vi "PMD Settings.vi"(0 "Visa In":refnum<visa-resource-name>, 1 "Zero?":refnum<vi>, 2 "PMD Settings In":T1 {"Averaging Rate" min=33 max=5000 step=1; "BWIn" items=["HIGH", "LOW"]; "Beam\nDiameter (mm)" min=1.0 max=9.0 step=0.5}, 3 "Error In":errorcluster, 4 "Range":i16 min=1 max=6 step=1) -> (5 "AUTO?":bool, 6 "Rng":string, 7 "Visa Out":refnum<visa-resource-name>, 8 "ZeroValue":dbl, 9 "PM Error log":string, 10 "error out":errorcluster)   [LabVIEW 2009]
panel:
  out "RANG_Val":dbl
  out "RANG_lbl":string
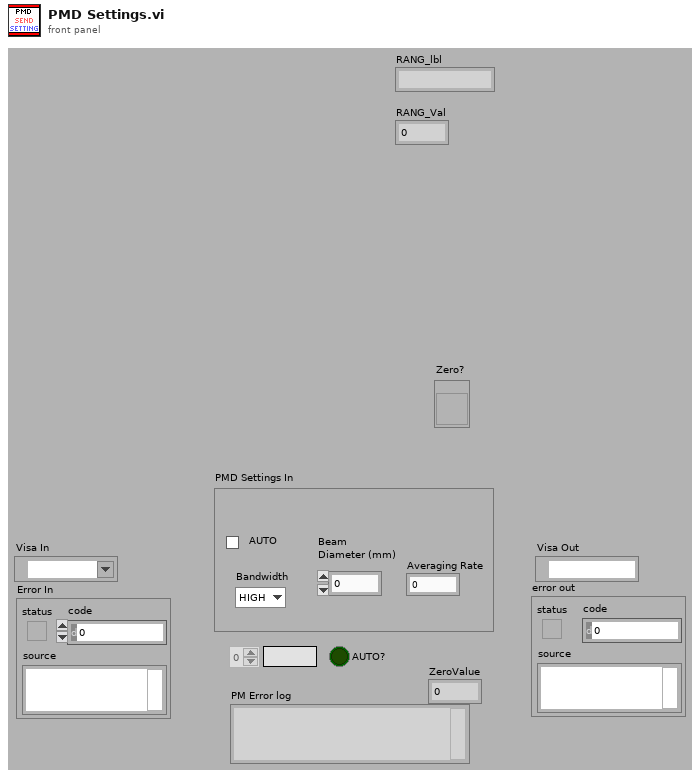
[diagram p1: front panel]
types:
  T1 = cluster{"Beam\nDiameter (mm)":dbl, "BWIn":u16, "Averaging Rate":i32, "AUTO":bool}
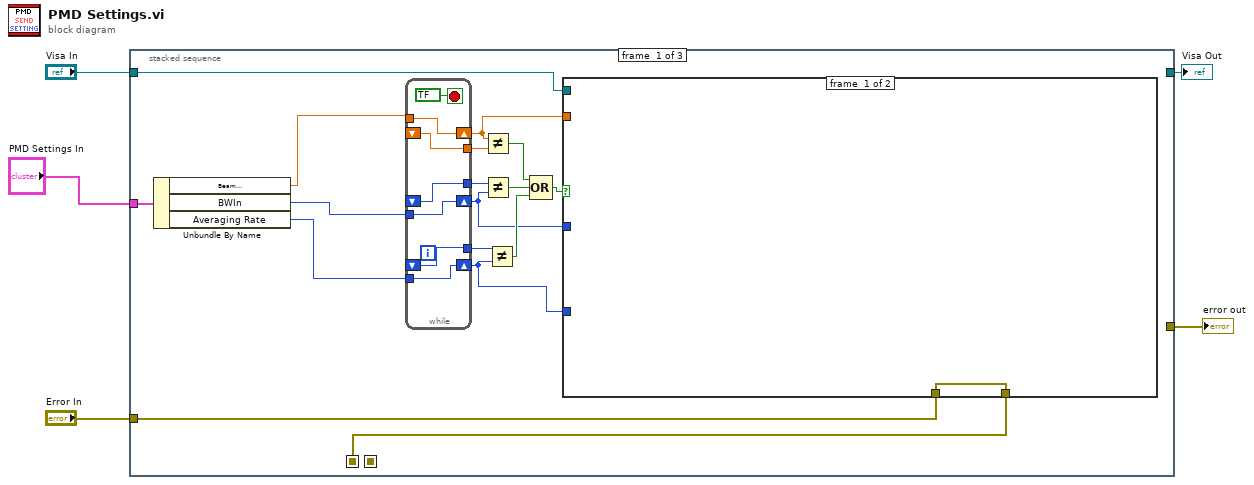
[diagram p0: block diagram]
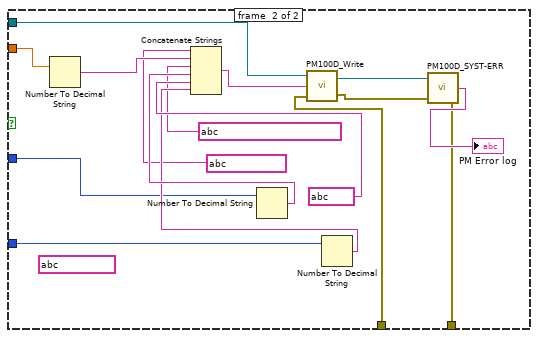
[diagram p2: hidden frame]
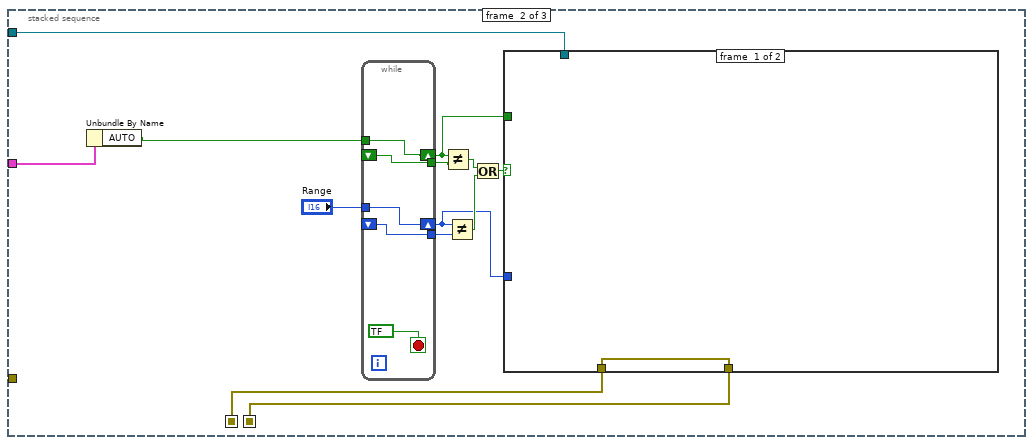
[diagram p3: hidden frame]
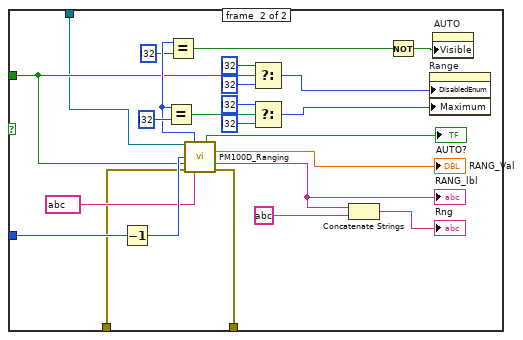
[diagram p4: hidden frame]
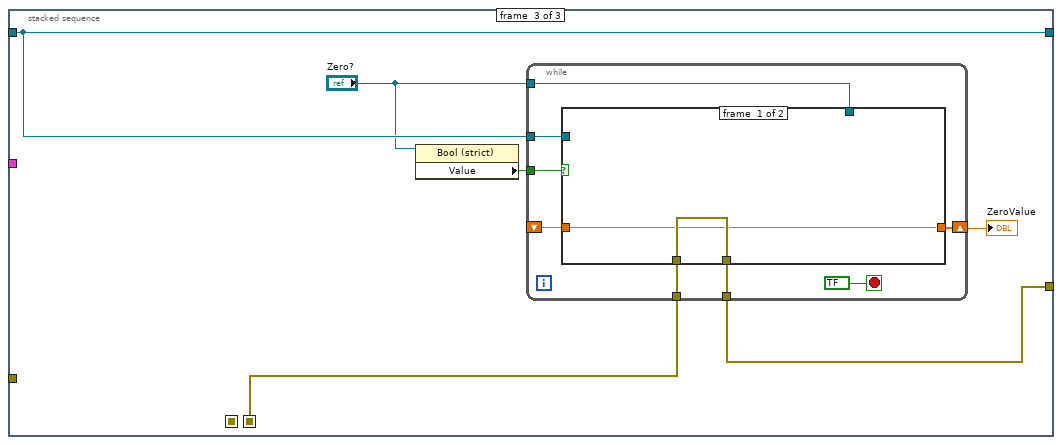
[diagram p5: hidden frame]
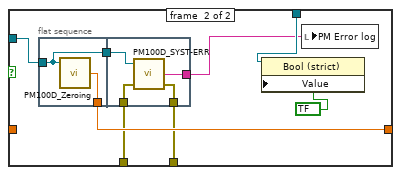
[diagram p6: hidden frame]
diagram:
  n1 = stacked-sequence {
    seq-local: [w12 _ _] -> [_ w51 _]
    seq-local: [_ w49 _] -> [_ _ w95]
    tunnel: "Error In" -> [w13 _ _]
    tunnel: "Visa In" -> [w11 w50 w93]
    tunnel: [_ _ w94] -> w3
    tunnel: [_ _ w93] -> w2
    tunnel: "PMD Settings In" -> [w9 w48 _]
    frame #0 {
      n2 = Unbundle By Name(w9) -> ("Beam\nDiameter (mm)"=w8:dbl, "BWIn"=w7:u16, "Averaging Rate"=w6:i32)
      n3 = while {
        shift-right: [w45] -> w14
        shift-left: _ -> [w44]
        shift-right: [w41] -> w15
        shift-left: _ -> [w40]
        shift-right: [w43] -> w10
        shift-left: _ -> [w42]
        tunnel: w8 -> [w45]
        tunnel: [w44] -> w22
        tunnel: w6 -> [w43]
        tunnel: [w42] -> w21
        tunnel: w7 -> [w41]
        tunnel: [w40] -> w16
        stop <- bool ? stop-if-true
      }
      n4 = Not Equal?(x=w14, y=w22) -> (x != y?=w18:bool)
      n5 = Not Equal?(x=w16, y=w15) -> (x != y?=w19:bool)
      n6 = Not Equal?(x=w21, y=w10) -> (x != y?=w20:bool)
      n7 = Compound Arithmetic op=OR(w18, w19, w20) -> (w17:bool)
      n8 = case shown="True" w17 {
        tunnel: w10 -> [_ w31]
        tunnel: w15 -> [_ w30]
        tunnel: w14 -> [_ w29]
        tunnel: w13 -> [w23 w28]
        tunnel: [w23 w27] -> w12
        tunnel: w11 -> [_ w26]
        frame #0 {
        }
        frame #1 {
          (unwired) string ? ("string")
          n9 = Number To Decimal String(number=w29) -> (decimal integer string=w32:string)  [unwired: 1 in]
          n10 = Number To Decimal String(number=w30) -> (decimal integer string=w36:string)  [unwired: 1 in]
          n11 = Number To Decimal String(number=w31) -> (decimal integer string=w33:string)  [unwired: 1 in]
          n12 = Concatenate Strings(string ? ("string"), w32, string ?, w36, string ? ("string"), w33) -> (w39:string)
          n13 = call "PM100D_Write.vi"("error in (no error)"=w28, "Command"=w39, "VISA in"=w26) -> ("error out"=w37:errorcluster, "VISA out"=w38:refnum<visa-resource-name>)
          n14 = call "PM100D_SYST-ERR.vi"("error out 2"=w37, "VISA In"=w38) -> ("error out"=w27:errorcluster, "Error"=→"PM Error log":string)  [unwired: 1 in, 1 out]
        }
      }
    }
    frame #1 {
      n15 = Unbundle By Name(w48) -> ("AUTO"=w47:bool)
      n16 = while {
        shift-right: [w87] -> w52
        shift-left: _ -> [w86]
        shift-right: [w89] -> w53
        shift-left: _ -> [w88]
        tunnel: w47 -> [w89]
        tunnel: [w88] -> w59
        tunnel: "Range" -> [w87]
        tunnel: [w86] -> w56
        stop <- bool ? stop-if-true
      }
      n17 = Not Equal?(x=w53, y=w59) -> (x != y?=w58:bool)
      n18 = Not Equal?(x=w52, y=w56) -> (x != y?=w55:bool)
      n19 = Or(x=w58, y=w55) -> (x .or. y?=w54:bool)
      n20 = case shown="True" w54 {
        tunnel: w53 -> [_ w67]
        tunnel: w52 -> [_ w66]
        tunnel: w50 -> [_ w64]
        tunnel: [w60 w62] -> w49
        tunnel: w51 -> [w60 w61]
        frame #0 {
        }
        frame #1 {
          n21 = Decrement(x=w66) -> (x-1=w74:i16)
          n22 = call "PM100D_Ranging.vi"("VISA in"=w64, "Index"=w74, "AUTO"=w67, "error in (no error)"=w61, "Unit"=string ?) -> ("SensType"=w73:i32, "AUTO?"=→"AUTO?":bool, "RANG_Val"=→"RANG_Val":dbl, "RANG_lbl"=w82:string, "error out"=w62:errorcluster)  [unwired: 3 in, 3 out]
          "RANG_lbl" <- w82
          n23 = Equal?(x=w73, y=i32 ?) -> (x = y?=w78:bool)
          n24 = Equal?(x=w73, y=i32 ?) -> (x = y?=w68:bool)
          n25 = Select(t=i32 ?, s=w67, f=i32 ?) -> (s? t:f=w80:i32)
          n26 = Select(t=i32 ?, s=w78, f=i32 ?) -> (s? t:f=w79:i32)
          n27 = Concatenate Strings(w82, string ?) -> (→"Rng":string)
          n28 = Not(x=w68) -> (.not. x?=w69:bool)
          n29 = property on="Range" class="DigNum (strict)"("DisabledEnum"=w80, "Maximum"=w79) -> ()  [unwired: 2 in, 2 out]
          n30 = property on="AUTO" class="Bool (strict)"("Visible"=w69) -> ()  [unwired: 2 in, 2 out]
        }
      }
    }
    frame #2 {
      n31 = property class="Bool (strict)"(reference="Zero?") -> ("Value"=w92:bool)  [unwired: 1 in, 2 out]
      n32 = while {
        tunnel: w95 -> [w103]
        tunnel: [w102] -> w94
        tunnel: w93 -> [w101]
        tunnel: w92 -> [w100]
        tunnel: "Zero?" -> [w99]
        shift-right: [w97] -> w90
        shift-left: _ -> [w96]
        stop <- bool ? stop-if-true
        n33 = case shown="True" w100 {
          tunnel: w101 -> [_ w113]
          tunnel: w103 -> [w105 w108]
          tunnel: [w105 w107] -> w102
          tunnel: w99 -> [_ w111]
          tunnel: [w104 w110] -> w97
          tunnel: w96 -> [w104 _]
          frame #0 {
          }
          frame #1 {
            n34 = flat-sequence {
              tunnel: w113 -> [w114]
              tunnel: [w115] -> w110
              tunnel: [w114] -> w106
              tunnel: [w119] -> w109
              tunnel: w108 -> [w118]
              tunnel: [w117] -> w107
              tunnel: w106 -> [w116]
              frame #0 {
                n35 = call "PM100D_Zeroing.vi"("VISA In"=w114) -> ("ZeroValue"=w115:dbl)  [unwired: 4 in]
              }
              frame #1 {
                n36 = call "PM100D_SYST-ERR.vi"("error out 2"=w118, "VISA In"=w116) -> ("error out"=w117:errorcluster, "Error"=w119:string)  [unwired: 1 in, 1 out]
              }
            }
            n37 = property class="Bool (strict)"(reference=w111, "Value"=bool ? ("Zero?")) -> ()  [unwired: 1 in, 2 out]
            n38 = local write "PM Error log"(w109) -> ()
          }
        }
      }
      "ZeroValue" <- w90
    }
  }
  "error out" <- w3
  "Visa Out" <- w2
